vi "Set String Message.vi"(7 "Format":string, 8 "error in (no error)":errorcluster, 9 "Value":string, 10 "Name":string, 11 "Message String in":refnum<class "Message String.lvclass">) -> (0 "error out":errorcluster, 3 "Message String out":refnum<class "Message String.lvclass">)   [LabVIEW 2016, in "Stream Mediator.lvlib" / "Message String.lvclass"]
doc: "--\nCopyright © 2017 Composed SystemsI All rights reserved.\n\nAuthor: Jon McBee <jon.mcbee@composed.io>\n\nThis library is provided \"AS IS\" ,WITHOUT WARRANTIES OR\nCONDITIONS OF ANY KIND, either express or implied.\n\nComposed Systems -- composed.io\n\nStream 0.0.1.1\nJon McBee - Composed Systems\nCopyright (c) 2017, Composed Systems"
uses:
  <userlib>/Composed Systems/Stream/Mediator/Classes/Message String/Message String.lvclass
  C:/Program Files (x86)/National Instruments/LabVIEW 2016/user.lib/Composed Systems/Stream/Mediator/Classes/Message Interface/Message Interface.lvclass
  <userlib>/Composed Systems/Stream/Mediator/Classes/Message String/Message String.lvclass/Message String.ctl
  <userlib>/Composed Systems/Stream/Mediator/Classes/Message Interface/Message Interface.lvclass
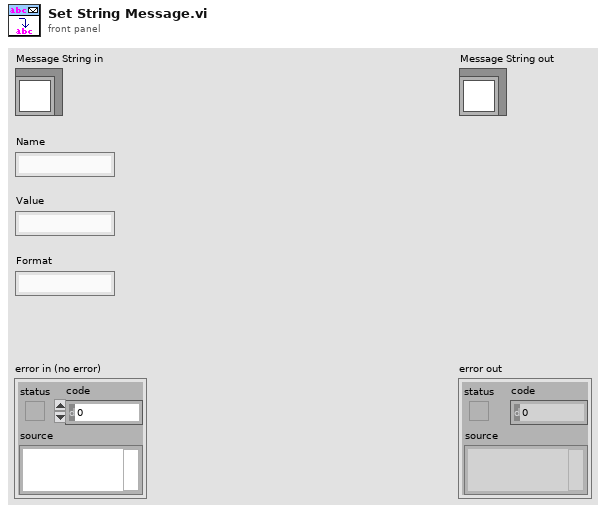
[diagram p1: front panel]
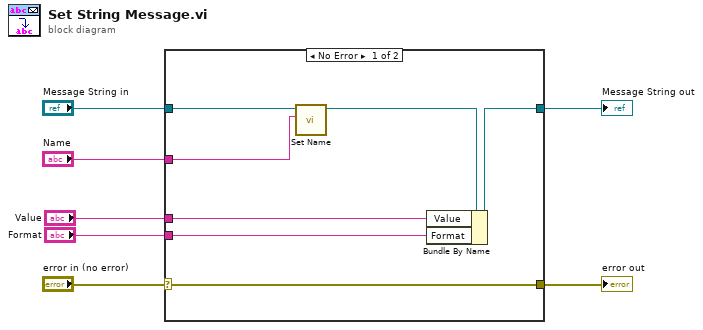
[diagram p0: block diagram]
diagram:
  n1 = case shown="No Error" "error in (no error)" {
    selector: "error in (no error)" -> [w14 w16]
    tunnel: [w14 w16] -> w6
    tunnel: [w13 w15] -> w4
    tunnel: "Message String in" -> [w10 w15]
    tunnel: "Value" -> [w12 _]
    tunnel: "Format" -> [w11 _]
    tunnel: "Name" -> [w8 _]
    frame No Error {
      n2 = call <userlib>:"Set Name.vi"("Name"=w8, "Message Interface in"=w10) -> ("Message Interface out"=w9:refnum<class "Message String.lvclass">)  [unwired: 8 in, 1 out]
      n3 = Bundle By Name(cluster=w9, "Value"=w12, "Format"=w11) -> (w13:refnum<class "Message String.lvclass">)
    }
    frame Error {
    }
  }
  "error out" <- w6
  "Message String out" <- w4
